vi "filter.delete.order.vi"(11 "filter.data in":T1 {"get.state"."v"."Quantity" format="%.0x"; "get.state"."v"."OrderId" format="%.0x"; "mem.cmd"."ord.2"."v"."Quantity" format="%016x"; "mem.cmd"."ord.2"."v"."OrderId" format="%016x"; "mem.cmd"."ord.1"."v"."Quantity" format="%016x"; "mem.cmd"."ord.1"."v"."OrderId" format="%016x"; "mem.cmd"."ticker"."v"."Symbol" format="%016x"; "mem.cmd"."order.slot.value"."Quantity" format="%016x"; "mem.cmd"."order.slot.value"."OrderId" format="%016x"; "debug"."v"."slot.3" format="%.0x"; "debug"."v"."slot.2" format="%.0x"; "debug"."v"."slot.1" format="%.0x"; "debug"."v"."slot.0" format="%.0x"; "Scratch"."OrderId" format="%016x"; "hash.2"."data.in" format="%.0x"; "hash.2"."crc32.out" format="%.0x"; "hash.1"."data.in" format="%.0x"; "hash.1"."crc32.out" format="%.0x"}) -> (3 "filter.data out":T1 {"get.state"."v"."Quantity" format="%.0x"; "get.state"."v"."OrderId" format="%.0x"; "mem.cmd"."ord.2"."v"."Quantity" format="%016x"; "mem.cmd"."ord.2"."v"."OrderId" format="%016x"; "mem.cmd"."ord.1"."v"."Quantity" format="%016x"; "mem.cmd"."ord.1"."v"."OrderId" format="%016x"; "mem.cmd"."ticker"."v"."Symbol" format="%016x"; "mem.cmd"."order.slot.value"."Quantity" format="%016x"; "mem.cmd"."order.slot.value"."OrderId" format="%016x"; "debug"."v"."slot.3" format="%.0x"; "debug"."v"."slot.2" format="%.0x"; "debug"."v"."slot.1" format="%.0x"; "debug"."v"."slot.0" format="%.0x"; "Scratch"."OrderId" format="%016x"; "hash.2"."data.in" format="%.0x"; "hash.2"."crc32.out" format="%.0x"; "hash.1"."data.in" format="%.0x"; "hash.1"."crc32.out" format="%.0x"})   [LabVIEW 2020]
uses:
  order.slot.ctl
  ticker.slot.ctl
  filter.memory.command.ctl
  filter.states.ctl
  filter.debug.slot.ctl
  filter.debug.ctl
  Market.Data.Common/fpga/orderbook.command.ctl
  Market.Data.Common/fpga/fpganow.common.fpga.lvlib
  Market.Data.Common/fpga/orderbook.command.type.ctl
  order.slot.hm.ctl
  order.slot.access.ctl
  ticker.slot.access.ctl
  filter.data.scratch.ctl
  filter.data.ctl
  filter.state.slot.ctl
  filter.state.ctl
  filter.hash.ctl
  Filter.lvclass
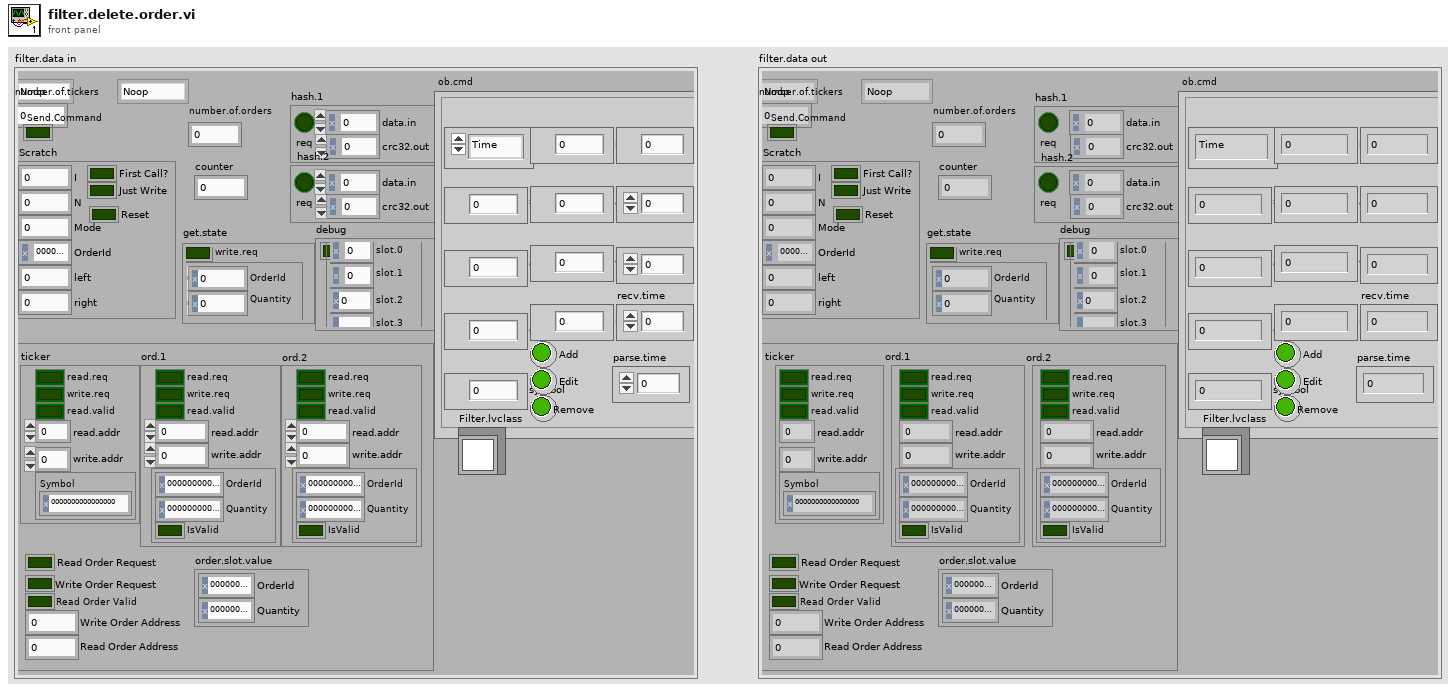
[diagram p1: front panel]
types:
  T1 = typedef "filter.data.ctl" = cluster{"filter.state":T2, "number.of.tickers":u32, "filter.saved.state":T2, "Send.Command":bool, "hash.1":T3, "hash.2":T3, "Scratch":T4, "debug":T5, "mem.cmd":T7, "get.state":T13, "ob.cmd":T15, "number.of.orders":u32, "Filter.lvclass":refnum<class "Filter.lvclass">, "counter":i16}
  T2 = typedef "filter.states.ctl" = enum16{"Noop", "Reset", "Debug", "Configuration", "Wait.for.Command", "Filter.Add", "Filter.Other", "Insert.Order", "Delete Order", "Get.State", "Get.Watchlist", "Get.Memory"}
  T3 = typedef "filter.hash.ctl" = cluster{"req":bool, "data.in":u64, "crc32.out":u32}
  T4 = typedef "filter.data.scratch.ctl" = cluster{"I":u32, "N":u32, "Mode":u32, "OrderId":u64, "First Call?":bool, "Just Write":bool, "left":u32, "right":u32, "Reset":bool}
  T5 = typedef "filter.debug.ctl" = cluster{"write":bool, "v":T6}
  T6 = typedef "filter.debug.slot.ctl" = cluster{"slot.0":u64, "slot.1":u64, "slot.2":u64, "slot.3":u64}
  T7 = typedef "filter.memory.command.ctl" = cluster{"Read Order Request":bool, "Write Order Request":bool, "Read Order Valid":bool, "Write Order Address":u32, "Read Order Address":u32, "order.slot.value":T8, "ticker":T9, "ord.1":T11, "ord.2":T11}
  T8 = typedef "order.slot.ctl" = cluster{"OrderId":u64, "Quantity":u64}
  T9 = typedef "ticker.slot.access.ctl" = cluster{"read.req":bool, "write.req":bool, "read.valid":bool, "read.addr":u32, "write.addr":u32, "v":T10}
  T10 = typedef "ticker.slot.ctl" = cluster{"Symbol":u64}
  T11 = typedef "order.slot.access.ctl" = cluster{"read.req":bool, "write.req":bool, "read.valid":bool, "read.addr":u32, "write.addr":u32, "v":T12}
  T12 = typedef "order.slot.hm.ctl" = cluster{"OrderId":u64, "Quantity":u64, "IsValid":bool}
  T13 = typedef "filter.state.ctl" = cluster{"write.req":bool, "v":T14}
  T14 = typedef "filter.state.slot.ctl" = cluster{"OrderId":u64, "Quantity":u64}
  T15 = typedef "fpganow.common.fpga.lvlib/orderbook.command.ctl" = cluster{"type":T16, "side":u8, "orderId ":u64, "quantity":u32, "symbol":u64, "price":u64, "executed.qty":u32, "canceled.qty":u32, "remaining.qty":u32, "seconds":u64, "nanoseconds":u64, "Add":bool, "Edit":bool, "Remove":bool, "seq no":u32, "recv.time":u64, "parse.time":u64}
  T16 = typedef "fpganow.common.fpga.lvlib/orderbook.command.type.ctl" = enum8{"Time", "AddOrder", "OrderExecuted", "OrderExecutedAtPrice", "ReduceSize", "ModifyOrder", "DeleteOrder", "Get.Everything", "Get.All.Orders", "Get.Top"}
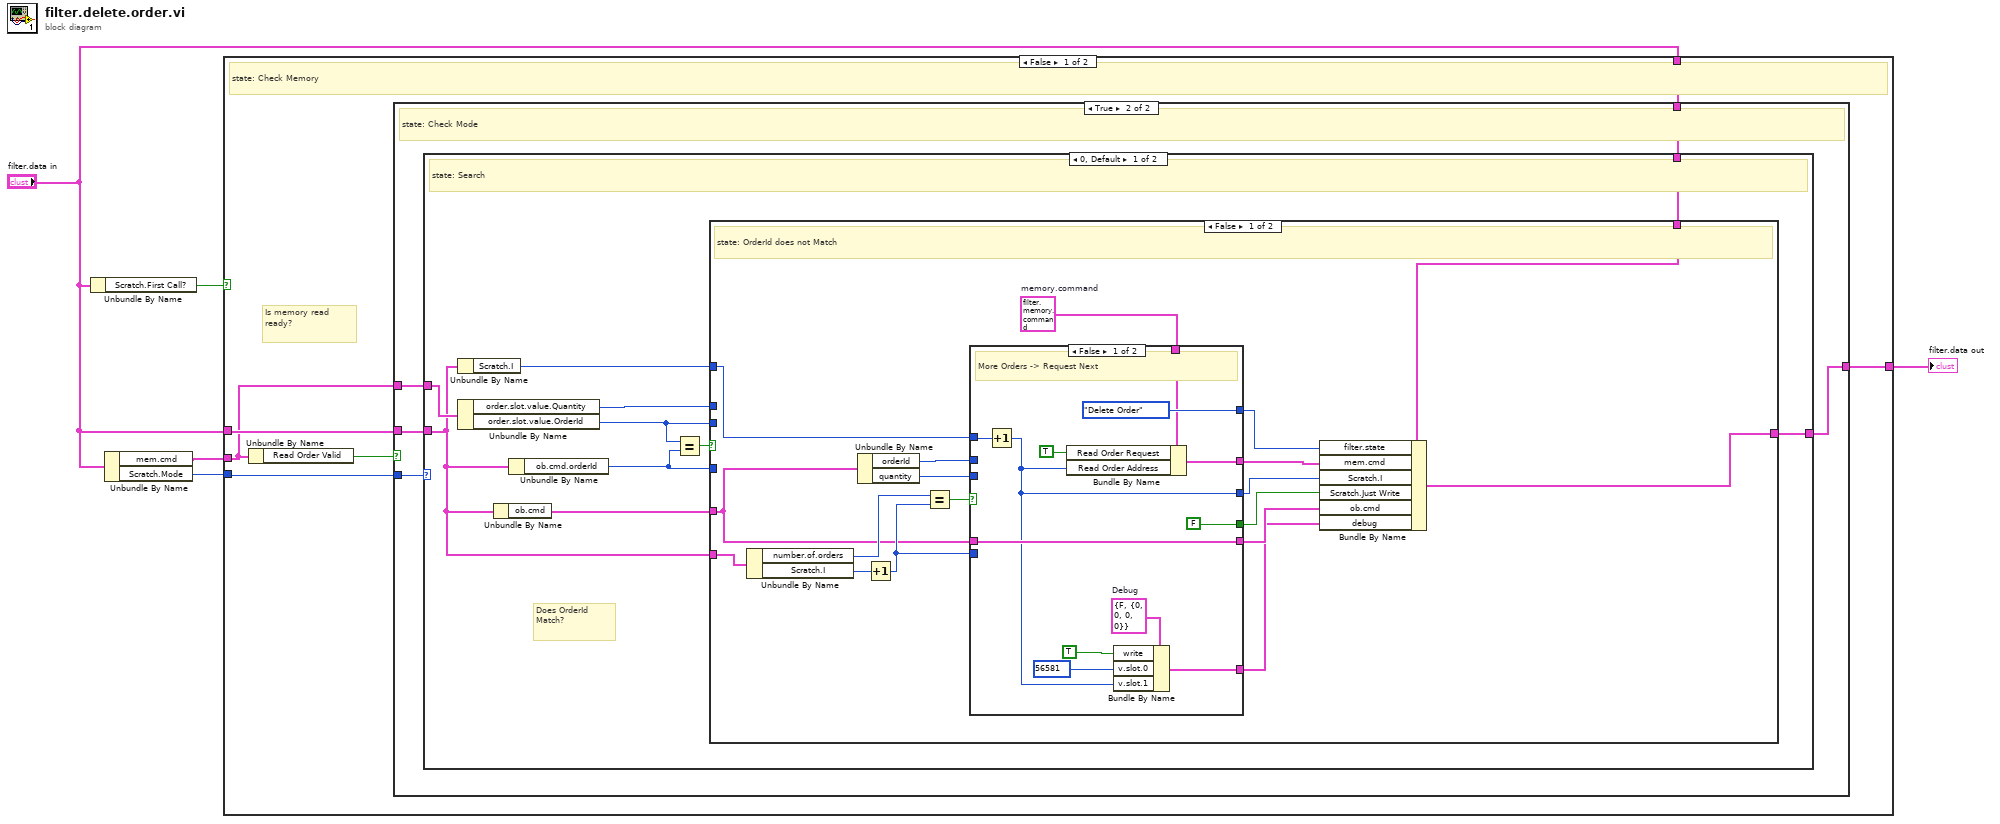
[diagram p0: block diagram]
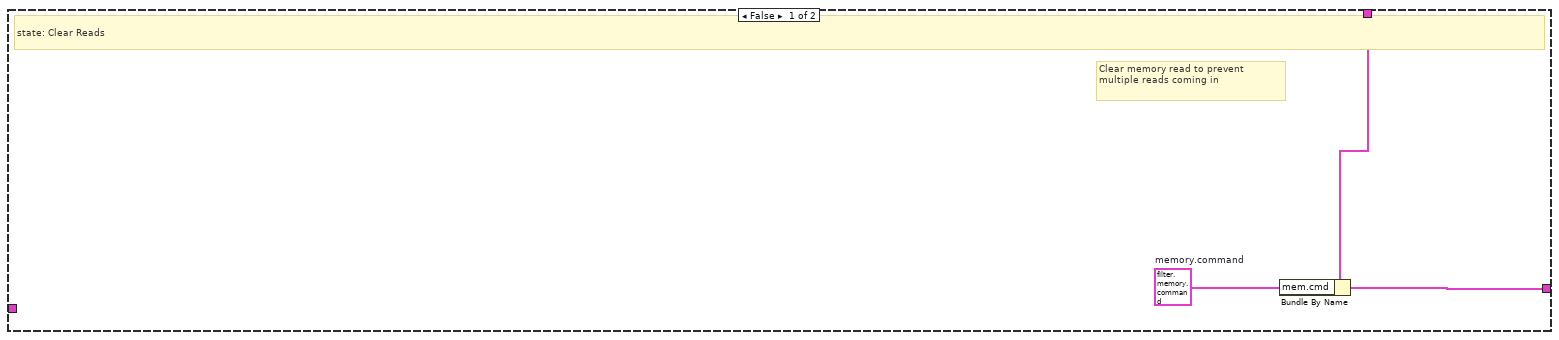
[diagram p2: hidden frame]
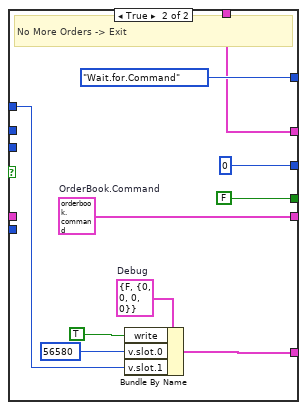
[diagram p3: hidden frame]
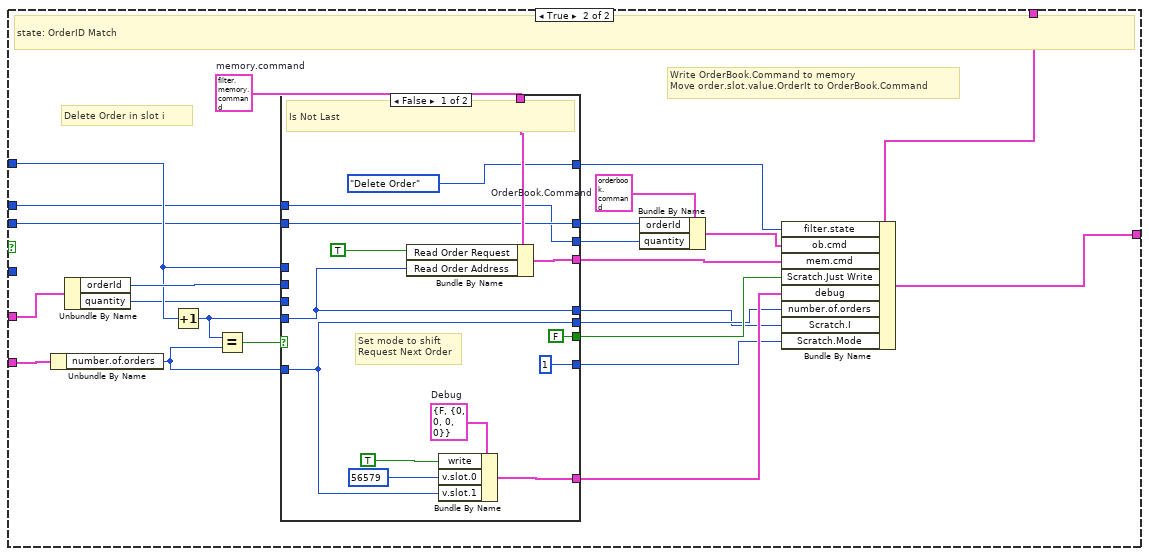
[diagram p4: hidden frame]
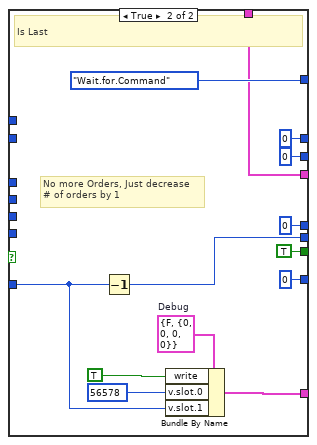
[diagram p5: hidden frame]
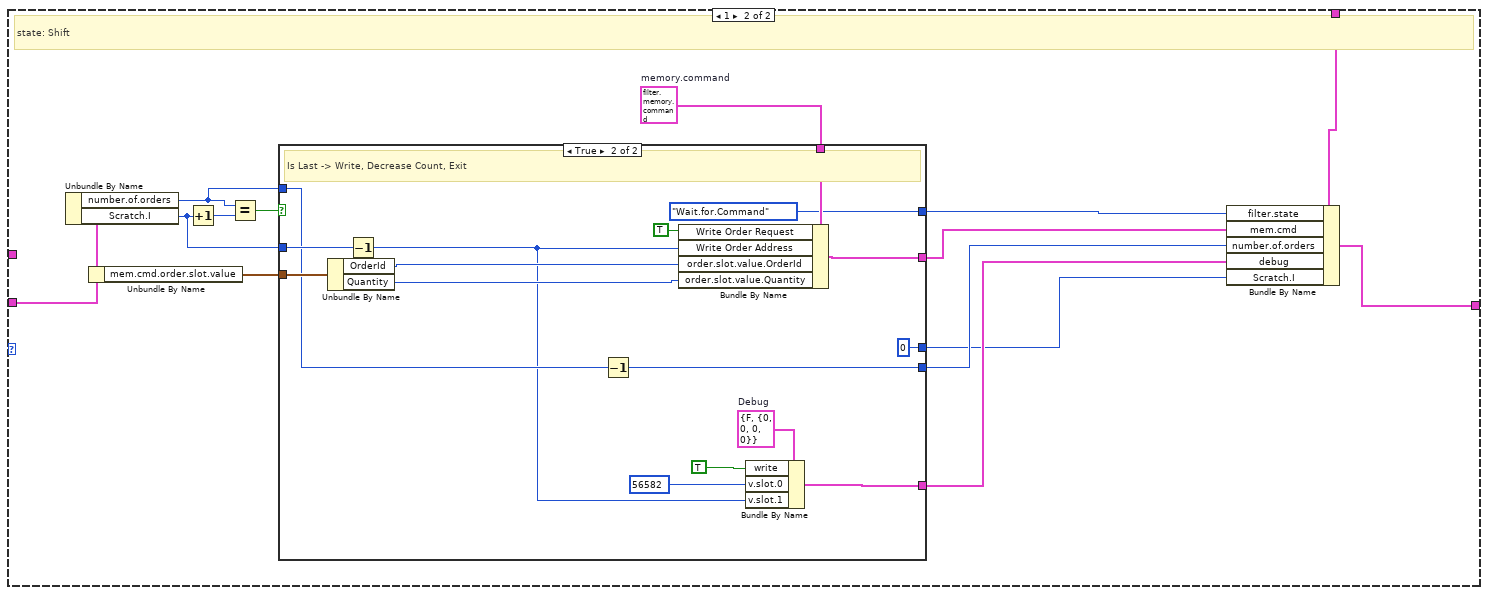
[diagram p6: hidden frame]
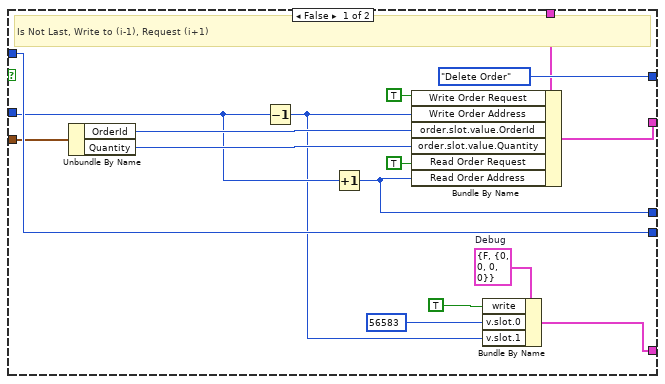
[diagram p7: hidden frame]
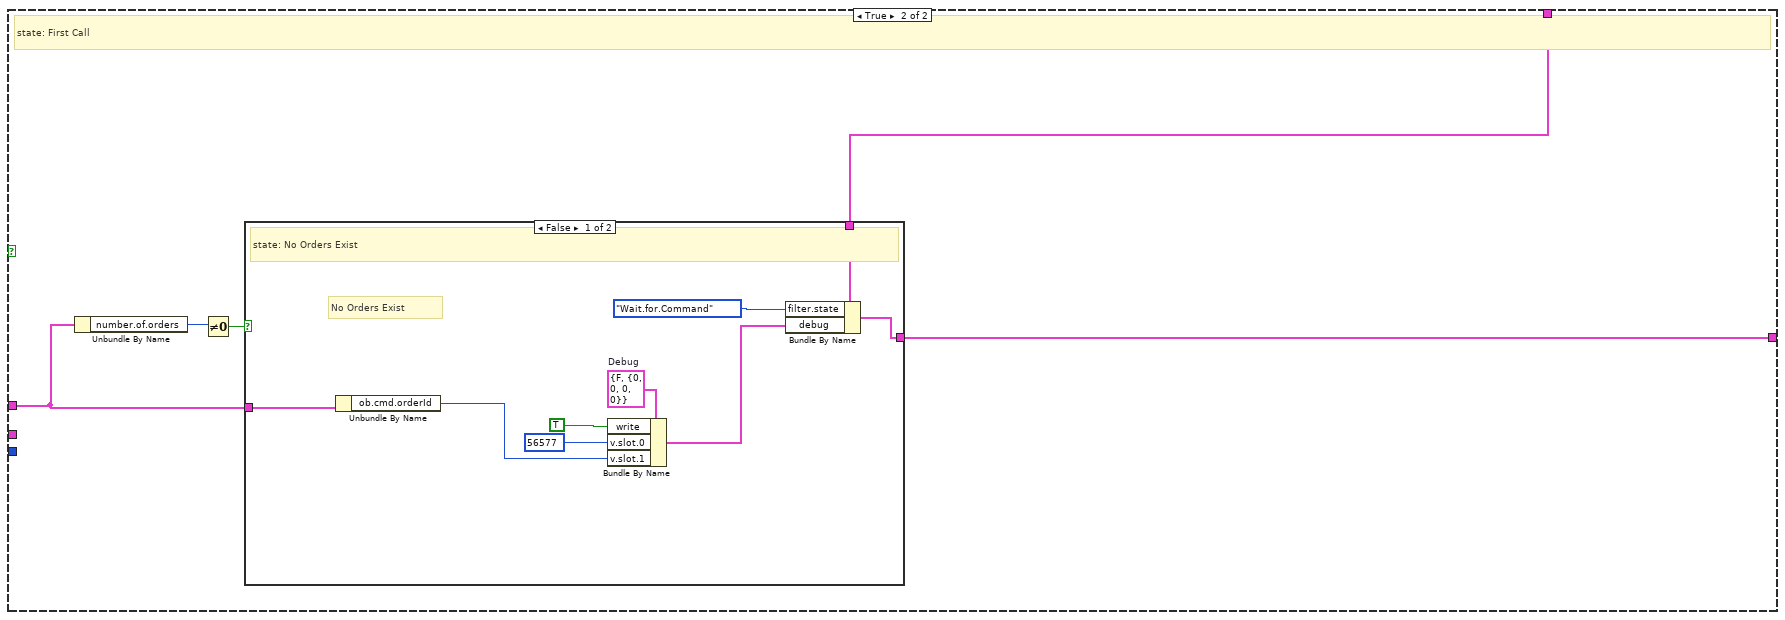
[diagram p8: hidden frame]
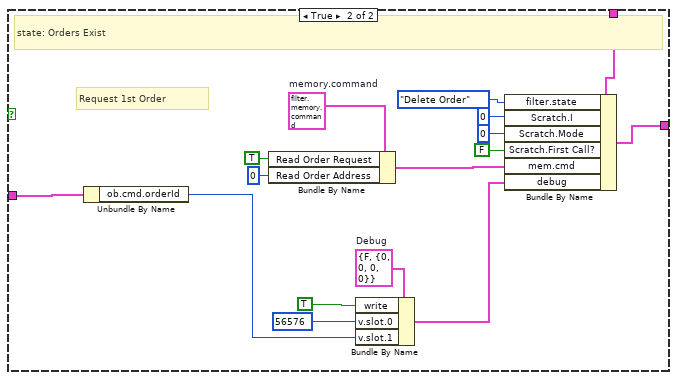
[diagram p9: hidden frame]
diagram:
  n1 = Unbundle By Name("filter.data in") -> ("Scratch.First Call?"=w2:bool)
  n2 = Unbundle By Name("filter.data in") -> ("mem.cmd"=w4:T7, "Scratch.Mode"=w1:u32)
  n3 = case shown="False" w2 {
    tunnel: "filter.data in" -> [w10 w168]
    tunnel: [w11 w167] -> w3
    tunnel: w4 -> [w8 _]
    tunnel: "filter.data in" -> [w9 w169]
    tunnel: w1 -> [w6 _]
    frame False {
      # "Is memory read\nready?"
      # "state: Check Memory"
      n4 = Unbundle By Name(w8) -> ("Read Order Valid"=w7:bool)
      n5 = case shown="True" w7 {
        tunnel: [w12 w17] -> w11
        tunnel: w10 -> [w14 w18]
        tunnel: w9 -> [_ w16]
        tunnel: w8 -> [_ w19]
        tunnel: w6 -> [_ w15]
        frame False {
          w13 = T7 {"Read Order Request"=FALSE, "Write Order Request"=FALSE, "Read Order Valid"=FALSE, "Write Order Address"=0, "Read Order Address"=0, "order.slot.value"={"OrderId"=0, "Quantity"=0}, "ticker"={"read.req"=FALSE, "write.req"=FALSE, "read.valid"=FALSE, "read.addr"=0, "write.addr"=0, "v"={"Symbol"=0}}, "ord.1"={"read.req"=FALSE, "write.req"=FALSE, "read.valid"=FALSE, "read.addr"=0, "write.addr"=0, "v"={"OrderId"=0, "Quantity"=0, "IsValid"=FALSE}}, "ord.2"={"read.req"=FALSE, "write.req"=FALSE, "read.valid"=FALSE, "read.addr"=0, "write.addr"=0, "v"={"OrderId"=0, "Quantity"=0, "IsValid"=FALSE}}}  # memory.command
          # "Clear memory read to prevent\nmultiple reads coming in"
          # "state: Clear Reads"
          n6 = Bundle By Name(cluster=w14, "mem.cmd"=w13) -> (w12:T1)
        }
        frame True {
          # "state: Check Mode"
          n7 = case shown="0, Default" w15 {
            tunnel: w19 -> [w29 _]
            tunnel: w18 -> [w27 w134]
            tunnel: [w26 w133] -> w17
            tunnel: w16 -> [w22 w127]
            frame 0, Default {
              # "Does OrderId\nMatch?"
              # "state: Search"
              n8 = Unbundle By Name(w22) -> ("Scratch.I"=w21:u32)
              n9 = Unbundle By Name(w29) -> ("order.slot.value.Quantity"=w20:u64, "order.slot.value.OrderId"=w24:u64)
              n10 = Unbundle By Name(w22) -> ("ob.cmd"=w25:T15)
              n11 = Unbundle By Name(w22) -> ("ob.cmd.orderId"=w23:u64)
              n12 = Equal?(x=w24, y=w23) -> (x = y?=w28:bool)
              n13 = case shown="False" w28 {
                tunnel: w27 -> [w46 w93]
                tunnel: [w47 w92] -> w26
                tunnel: w25 -> [w32 w87]
                tunnel: w22 -> [w45 w84]
                tunnel: w24 -> [_ w79]
                tunnel: w21 -> [w37 w85]
                tunnel: w23 -> [_ _]
                tunnel: w20 -> [_ w72]
                frame False {
                  w39 = T7 {"Read Order Request"=FALSE, "Write Order Request"=FALSE, "Read Order Valid"=FALSE, "Write Order Address"=0, "Read Order Address"=0, "order.slot.value"={"OrderId"=0, "Quantity"=0}, "ticker"={"read.req"=FALSE, "write.req"=FALSE, "read.valid"=FALSE, "read.addr"=0, "write.addr"=0, "v"={"Symbol"=0}}, "ord.1"={"read.req"=FALSE, "write.req"=FALSE, "read.valid"=FALSE, "read.addr"=0, "write.addr"=0, "v"={"OrderId"=0, "Quantity"=0, "IsValid"=FALSE}}, "ord.2"={"read.req"=FALSE, "write.req"=FALSE, "read.valid"=FALSE, "read.addr"=0, "write.addr"=0, "v"={"OrderId"=0, "Quantity"=0, "IsValid"=FALSE}}}  # memory.command
                  # "state: OrderId does not Match"
                  n14 = Unbundle By Name(w45) -> ("number.of.orders"=w36:u32, "Scratch.I"=w44:u32)
                  n15 = Unbundle By Name(w32) -> ("orderId"=w38:u64, "quantity"=w30:u32)
                  n16 = Increment(x=w44) -> (x+1=w41:u32)
                  n17 = Equal?(x=w36, y=w41) -> (x = y?=w42:bool)
                  n18 = case shown="False" w42 {
                    tunnel: [w59 w68] -> w43
                    tunnel: w41 -> [_ _]
                    tunnel: [filter.states."Delete Order" ("filter.state") filter.states."Wait.for.Command" ("filter.state")] -> w40
                    tunnel: w39 -> [w56 w68]
                    tunnel: w38 -> [_ _]
                    tunnel: w37 -> [w50 w67]
                    tunnel: [w48 u32 0] -> w35
                    tunnel: [FALSE ("Scratch.Just Write") FALSE ("Scratch.Just Write")] -> w34
                    tunnel: [w54 w64] -> w33
                    tunnel: w32 -> [w54 _]
                    tunnel: [w52 w62] -> w31
                    tunnel: w30 -> [_ _]
                    frame False {
                      w53 = T5 {"write"=FALSE, "v"={"slot.0"=0, "slot.1"=0, "slot.2"=0, "slot.3"=0}}  # Debug
                      # "More Orders -> Request Next"
                      n19 = Increment(x=w50) -> (x+1=w48:u32)
                      n20 = Bundle By Name(cluster=w56, "Read Order Request"=TRUE ("Read.Request"), "Read Order Address"=w48) -> (w59:T7)
                      n21 = Bundle By Name(cluster=w53, "write"=TRUE ("Write.to.Debug"), "v.slot.0"=u64 56581 ("debug.slot.OrderId"), "v.slot.1"=w48) -> (w52:T5)
                    }
                    frame True {
                      w63 = T5 {"write"=FALSE, "v"={"slot.0"=0, "slot.1"=0, "slot.2"=0, "slot.3"=0}}  # Debug
                      w64 = T15 {"type"=enum."Time", "side"=0, "orderId "=0, "quantity"=0, "symbol"=0, "price"=0, "executed.qty"=0, "canceled.qty"=0, "remaining.qty"=0, "seconds"=0, "nanoseconds"=0, "Add"=FALSE, "Edit"=FALSE, "Remove"=FALSE, "seq no"=0, "recv.time"=0, "parse.time"=0}  # OrderBook.Command
                      # "No More Orders -> Exit"
                      n22 = Bundle By Name(cluster=w63, "write"=TRUE ("Write.to.Debug"), "v.slot.0"=u64 56580 ("debug.slot.OrderId"), "v.slot.1"=w67) -> (w62:T5)
                    }
                  }
                  n23 = Bundle By Name(cluster=w46, "filter.state"=w40, "mem.cmd"=w43, "Scratch.I"=w35, "Scratch.Just Write"=w34, "ob.cmd"=w33, "debug"=w31) -> (w47:T1)
                }
                frame True {
                  w90 = T15 {"type"=enum."Time", "side"=0, "orderId "=0, "quantity"=0, "symbol"=0, "price"=0, "executed.qty"=0, "canceled.qty"=0, "remaining.qty"=0, "seconds"=0, "nanoseconds"=0, "Add"=FALSE, "Edit"=FALSE, "Remove"=FALSE, "seq no"=0, "recv.time"=0, "parse.time"=0}  # OrderBook.Command
                  w89 = T7 {"Read Order Request"=FALSE, "Write Order Request"=FALSE, "Read Order Valid"=FALSE, "Write Order Address"=0, "Read Order Address"=0, "order.slot.value"={"OrderId"=0, "Quantity"=0}, "ticker"={"read.req"=FALSE, "write.req"=FALSE, "read.valid"=FALSE, "read.addr"=0, "write.addr"=0, "v"={"Symbol"=0}}, "ord.1"={"read.req"=FALSE, "write.req"=FALSE, "read.valid"=FALSE, "read.addr"=0, "write.addr"=0, "v"={"OrderId"=0, "Quantity"=0, "IsValid"=FALSE}}, "ord.2"={"read.req"=FALSE, "write.req"=FALSE, "read.valid"=FALSE, "read.addr"=0, "write.addr"=0, "v"={"OrderId"=0, "Quantity"=0, "IsValid"=FALSE}}}  # memory.command
                  # "Write OrderBook.Command to memory\nMove order.slot.value.OrderIt to OrderBook.Command"
                  # "Delete Order in slot i"
                  # "state: OrderID Match"
                  n24 = Unbundle By Name(w84) -> ("number.of.orders"=w76:u32)
                  n25 = Unbundle By Name(w87) -> ("orderId"=w86:u64, "quantity"=w74:u32)
                  n26 = Increment(x=w85) -> (x+1=w83:u32)
                  n27 = Equal?(x=w83, y=w76) -> (x = y?=w82:bool)
                  n28 = case shown="False" w82 {
                    tunnel: w89 -> [w107 w111]
                    tunnel: [w106 w111] -> w88
                    tunnel: w86 -> [_ _]
                    tunnel: w85 -> [_ _]
                    tunnel: w83 -> [w98 _]
                    tunnel: [w104 u64 0 ("OrderId")] -> w81
                    tunnel: w79 -> [w104 _]
                    tunnel: [FALSE ("Scratch.Just Write") TRUE ("Scratch.Just Write")] -> w80
                    tunnel: [w99 w116] -> w78
                    tunnel: [w96 w114] -> w77
                    tunnel: w76 -> [w96 w113]
                    tunnel: [w98 u32 0] -> w75
                    tunnel: w74 -> [_ _]
                    tunnel: [w97 u64 0 ("Quantity")] -> w73
                    tunnel: w72 -> [w97 _]
                    tunnel: [filter.states."Delete Order" ("filter.state") filter.states."Wait.for.Command" ("filter.state")] -> w71
                    tunnel: [u32 1 ("Scratch.Mode") u32 0 ("Scratch.Mode")] -> w70
                    frame False {
                      w102 = T5 {"write"=FALSE, "v"={"slot.0"=0, "slot.1"=0, "slot.2"=0, "slot.3"=0}}  # Debug
                      # "Set mode to shift\nRequest Next Order"
                      # "Is Not Last"
                      n29 = Bundle By Name(cluster=w107, "Read Order Request"=TRUE ("Read Order\nRequest"), "Read Order Address"=w98) -> (w106:T7)
                      n30 = Bundle By Name(cluster=w102, "write"=TRUE ("Write.to.Debug"), "v.slot.0"=u64 56579 ("debug.slot.Ticker"), "v.slot.1"=w96) -> (w99:T5)
                    }
                    frame True {
                      w119 = T5 {"write"=FALSE, "v"={"slot.0"=0, "slot.1"=0, "slot.2"=0, "slot.3"=0}}  # Debug
                      # "No more Orders, Just decrease\n# of orders by 1"
                      # "Is Last"
                      n31 = Decrement(x=w113) -> (x-1=w114:u32)
                      n32 = Bundle By Name(cluster=w119, "write"=TRUE ("Write.to.Debug"), "v.slot.0"=u64 56578 ("debug.slot.Ticker"), "v.slot.1"=w113) -> (w116:T5)
                    }
                  }
                  n33 = Bundle By Name(cluster=w90, "orderId"=w81, "quantity"=w73) -> (w91:T15)
                  n34 = Bundle By Name(cluster=w93, "filter.state"=w71, "ob.cmd"=w91, "mem.cmd"=w88, "Scratch.Just Write"=w80, "debug"=w78, "number.of.orders"=w77, "Scratch.I"=w75, "Scratch.Mode"=w70) -> (w92:T1)
                }
              }
            }
            frame 1 {
              w131 = T7 {"Read Order Request"=FALSE, "Write Order Request"=FALSE, "Read Order Valid"=FALSE, "Write Order Address"=0, "Read Order Address"=0, "order.slot.value"={"OrderId"=0, "Quantity"=0}, "ticker"={"read.req"=FALSE, "write.req"=FALSE, "read.valid"=FALSE, "read.addr"=0, "write.addr"=0, "v"={"Symbol"=0}}, "ord.1"={"read.req"=FALSE, "write.req"=FALSE, "read.valid"=FALSE, "read.addr"=0, "write.addr"=0, "v"={"OrderId"=0, "Quantity"=0, "IsValid"=FALSE}}, "ord.2"={"read.req"=FALSE, "write.req"=FALSE, "read.valid"=FALSE, "read.addr"=0, "write.addr"=0, "v"={"OrderId"=0, "Quantity"=0, "IsValid"=FALSE}}}  # memory.command
              # "state: Shift"
              n35 = Unbundle By Name(w127) -> ("number.of.orders"=w124:u32, "Scratch.I"=w129:u32)
              n36 = Unbundle By Name(w127) -> ("mem.cmd.order.slot.value"=w126:T8)
              n37 = Increment(x=w129) -> (x+1=w130:u32)
              n38 = Equal?(x=w124, y=w130) -> (x = y?=w132:bool)
              n39 = case shown="True" w132 {
                tunnel: w131 -> [w148 w166]
                tunnel: w129 -> [w137 w164]
                tunnel: [w147 w163] -> w128
                tunnel: w126 -> [w141 w162]
                tunnel: [w146 w158] -> w125
                tunnel: w124 -> [w146 w159]
                tunnel: [filter.states."Delete Order" ("filter.state") filter.states."Wait.for.Command" ("filter.state")] -> w123
                tunnel: [w142 w153] -> w122
                tunnel: [w135 u32 0] -> w121
                frame False {
                  w145 = T5 {"write"=FALSE, "v"={"slot.0"=0, "slot.1"=0, "slot.2"=0, "slot.3"=0}}  # Debug
                  # "Is Not Last, Write to (i-1), Request (i+1)"
                  n40 = Unbundle By Name(w141) -> ("OrderId"=w140:u64, "Quantity"=w139:u64)
                  n41 = Decrement(x=w137) -> (x-1=w136:u32)
                  n42 = Increment(x=w137) -> (x+1=w135:u32)
                  n43 = Bundle By Name(cluster=w148, "Write Order Request"=TRUE ("Write Order\nRequest"), "Write Order Address"=w136, "order.slot.value.OrderId"=w140, "order.slot.value.Quantity"=w139, "Read Order Request"=TRUE ("Read Order\nRequest"), "Read Order Address"=w135) -> (w147:T7)
                  n44 = Bundle By Name(cluster=w145, "write"=TRUE ("Write.to.Debug"), "v.slot.0"=u64 56583 ("debug.slot.OrderId"), "v.slot.1"=w136) -> (w142:T5)
                }
                frame True {
                  w154 = T5 {"write"=FALSE, "v"={"slot.0"=0, "slot.1"=0, "slot.2"=0, "slot.3"=0}}  # Debug
                  # "Is Last -> Write, Decrease Count, Exit"
                  n45 = Unbundle By Name(w162) -> ("OrderId"=w161:u64, "Quantity"=w160:u64)
                  n46 = Decrement(x=w164) -> (x-1=w152:u32)
                  n47 = Decrement(x=w159) -> (x-1=w158:u32)
                  n48 = Bundle By Name(cluster=w166, "Write Order Request"=TRUE ("Write Order\nRequest"), "Write Order Address"=w152, "order.slot.value.OrderId"=w161, "order.slot.value.Quantity"=w160) -> (w163:T7)
                  n49 = Bundle By Name(cluster=w154, "write"=TRUE ("Write.to.Debug"), "v.slot.0"=u64 56582 ("debug.slot.OrderId"), "v.slot.1"=w152) -> (w153:T5)
                }
              }
              n50 = Bundle By Name(cluster=w134, "filter.state"=w123, "mem.cmd"=w128, "number.of.orders"=w125, "debug"=w122, "Scratch.I"=w121) -> (w133:T1)
            }
          }
        }
      }
    }
    frame True {
      # "state: First Call"
      n51 = Unbundle By Name(w169) -> ("number.of.orders"=w171:u32)
      n52 = Not Equal To 0?(x=w171) -> (x != 0?=w170:bool)
      n53 = case shown="False" w170 {
        tunnel: w169 -> [w175 w184]
        tunnel: w168 -> [w173 w182]
        tunnel: [w172 w181] -> w167
        frame False {
          w179 = T5 {"write"=FALSE, "v"={"slot.0"=0, "slot.1"=0, "slot.2"=0, "slot.3"=0}}  # Debug
          # "No Orders Exist"
          # "state: No Orders Exist"
          n54 = Unbundle By Name(w175) -> ("ob.cmd.orderId"=w177:u64)
          n55 = Bundle By Name(cluster=w179, "write"=TRUE ("Write.to.Debug"), "v.slot.0"=u64 56577 ("debug.slot.Ticker"), "v.slot.1"=w177) -> (w174:T5)
          n56 = Bundle By Name(cluster=w173, "filter.state"=filter.states."Wait.for.Command", "debug"=w174) -> (w172:T1)
        }
        frame True {
          w188 = T5 {"write"=FALSE, "v"={"slot.0"=0, "slot.1"=0, "slot.2"=0, "slot.3"=0}}  # Debug
          w195 = T7 {"Read Order Request"=FALSE, "Write Order Request"=FALSE, "Read Order Valid"=FALSE, "Write Order Address"=0, "Read Order Address"=0, "order.slot.value"={"OrderId"=0, "Quantity"=0}, "ticker"={"read.req"=FALSE, "write.req"=FALSE, "read.valid"=FALSE, "read.addr"=0, "write.addr"=0, "v"={"Symbol"=0}}, "ord.1"={"read.req"=FALSE, "write.req"=FALSE, "read.valid"=FALSE, "read.addr"=0, "write.addr"=0, "v"={"OrderId"=0, "Quantity"=0, "IsValid"=FALSE}}, "ord.2"={"read.req"=FALSE, "write.req"=FALSE, "read.valid"=FALSE, "read.addr"=0, "write.addr"=0, "v"={"OrderId"=0, "Quantity"=0, "IsValid"=FALSE}}}  # memory.command
          # "Request 1st Order"
          # "state: Orders Exist"
          n57 = Unbundle By Name(w184) -> ("ob.cmd.orderId"=w186:u64)
          n58 = Bundle By Name(cluster=w195, "Read Order Request"=TRUE ("Read.Request"), "Read Order Address"=u32 0 ("Read Order\nAddress")) -> (w190:T7)
          n59 = Bundle By Name(cluster=w188, "write"=TRUE ("Write.to.Debug"), "v.slot.0"=u64 56576 ("debug.slot.Ticker"), "v.slot.1"=w186) -> (w183:T5)
          n60 = Bundle By Name(cluster=w182, "filter.state"=filter.states."Delete Order", "Scratch.I"=u32 0, "Scratch.Mode"=u32 0, "Scratch.First Call?"=FALSE, "mem.cmd"=w190, "debug"=w183) -> (w181:T1)
        }
      }
    }
  }
  "filter.data out" <- w3
